vi "Autonomous Independent.vi"   [LabVIEW 2019]
doc: "This VI is called when autonomous begins, and will automatically be terminated when autonomous ends. You can carry out timed or sensor driven robot movement independently without needing to return to the caller."
uses:
  <vilib>/Rock Robotics/WPI/Utilities/WPI_GetSetVariantRefNum.vi
  <vilib>/Rock Robotics/Network Tables/NT Read String.vi
  <vilib>/Rock Robotics/Network Tables/NT Write Numeric Array.vi
  Robot Global Data.vi
panel:
  # "Be sure to right-click and choose Data Operations>>Make Current Value default if you want to save the array values with the VI"
types:
  T1 = typedef "WPI_JoystickDevRef.ctl" = cluster{"Device":T2}
  T2 = typedef "WPI_JoystickDeviceEnum.ctl" = enum16{"USB 0", "USB 1", "USB 2", "USB 3", "USB 4", "USB 5"}
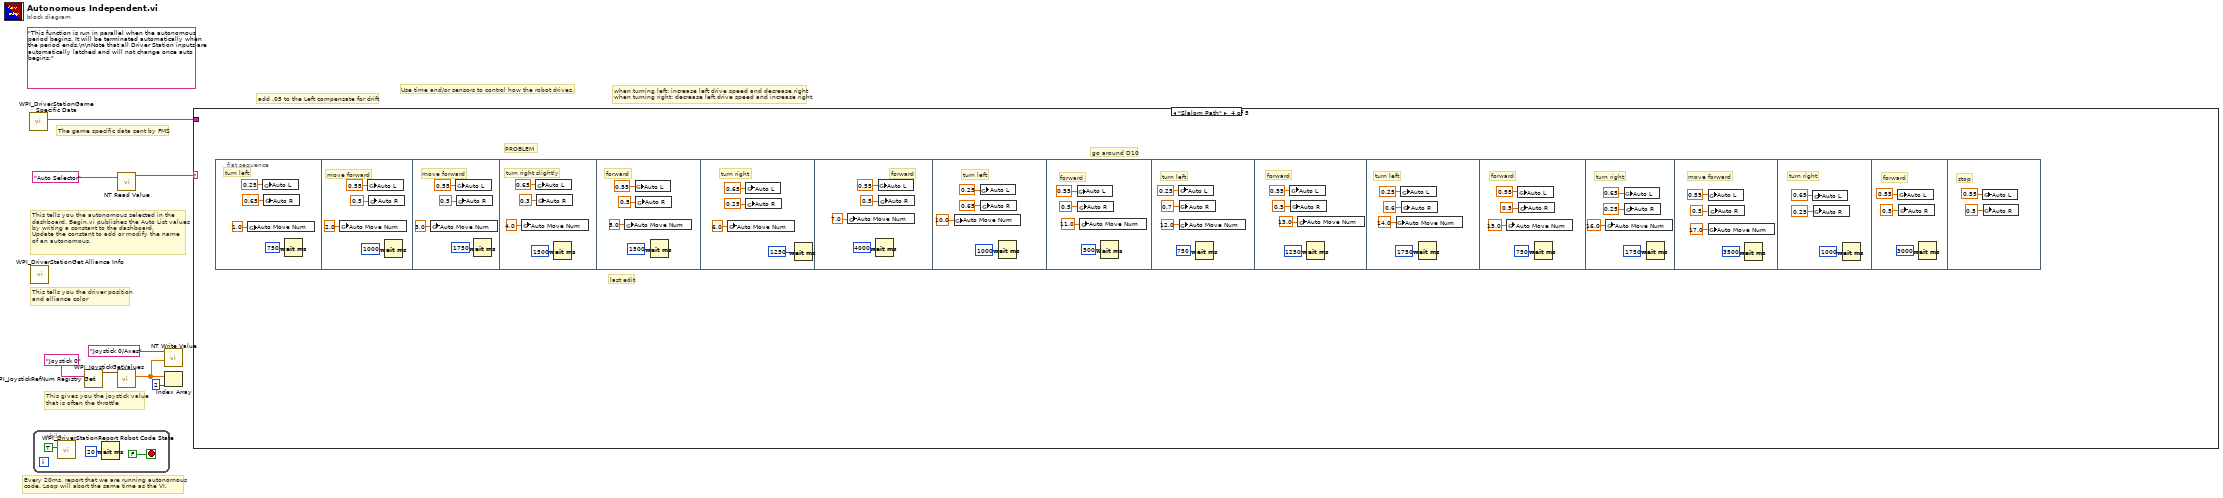
[diagram p0: block diagram]
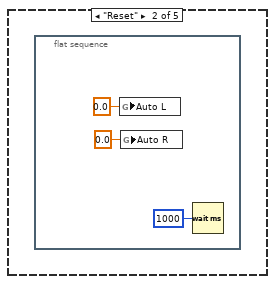
[diagram p3: hidden frame]
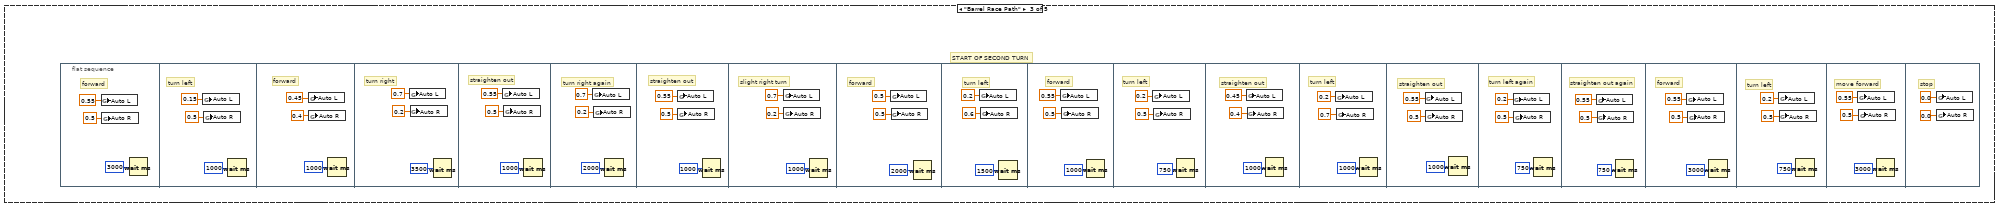
[diagram p4: hidden frame]
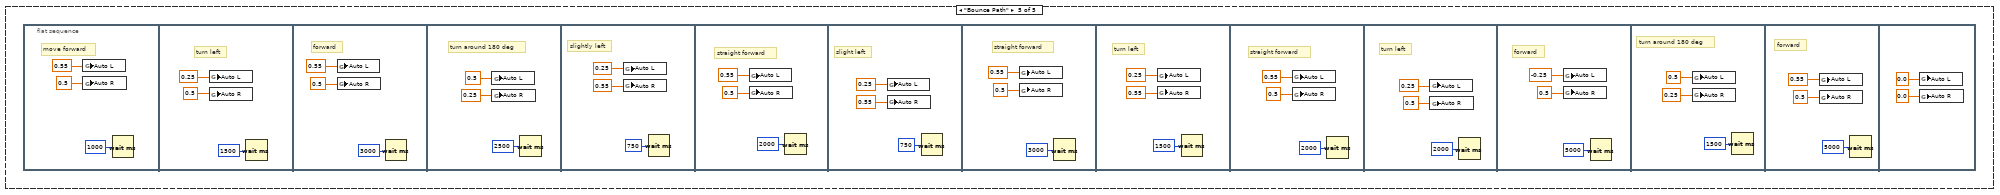
[diagram p5: hidden frame]
diagram:
  (unwired) "This function is run in parallel when the autonomous period begins. It will be terminated automatically when the period ends.\n\nNote that all Driver Station inputs are automatically latched and will not change once auto begins."
  # "add .05 to the Left compensate for drift"
  # "when turning left: increase left drive speed and decrease right\nwhen turning right: decrease left drive speed and increase right"
  # "The game specific data sent by FMS"
  # "This tells you the autonomous selected in the \ndashboard. Begin.vi publishes the Auto List values\nby writing a constant to the dashboard.\nUpdate the constant to add or modify the name\nof an autonomous."
  # "Every 20ms, report that we are running autonomous\ncode. Loop will abort the same time as the VI."
  # "This gives you the joystick value\nthat is often the throttle"
  # "Use time and/or sensors to control how the robot drives."
  # "This tells you the driver position\nand alliance color"
  n1 = call <vilib>:"WPI_DriverStationGame Specific Data.vi"() -> ("Game Specific Data"=w1:string)  [unwired: 11 in]
  n2 = call <vilib>:"WPI_DriverStationGet Alliance Info.vi"() -> ()  [unwired: 12 out]
  n3 = while {
    stop <- FALSE stop-if-true
    n4 = call <vilib>:"WPI_DriverStationReport Robot Code State.vi"("Autonomous"=TRUE) -> ()  [unwired: 10 in, 1 out]
    n5 = Wait (ms)(milliseconds to wait=u32 20) -> ()  [unwired: 1 out]
  }
  n6 = call <vilib>:"WPI_JoystickRefNum Registry Get.vi"("refnum name"="Joystick 0") -> ("JoystickDevRef"=w7:T1)  [unwired: 1 in, 9 out]
  n7 = call <vilib>:"WPI_JoystickGetValues.vi"("JoystickDevRef"=w7) -> ("Axes"=w3:dbl[])  [unwired: 6 in, 4 out]
  n8 = call-poly <vilib>:"NT Read Value.vi"("Name"="Auto Selector") -> ("String"=w4:string)  [unwired: 9 in, 1 out]
  n9 = call-poly <vilib>:"NT Write Value.vi"("Numeric Array"=w3, "Name"="Joystick 0/Axes") -> ()  [unwired: 9 in, 1 out]
  n10 = Index Array(array=w3, index=2) -> ()  [unwired: 1 out]
  n11 = case shown="\"Slalom Path\"" w4 {
    tunnel: w1 -> [_ _ _ _ _]
    frame Default {
      # "You can put your main auto here, or you can right-click on the case and make any\nother frame be the default case."
      # "This is the frame that will execute if no selection is made, or if it is not recognized"
    }
    frame "Reset" {
      n12 = flat-sequence {
        frame #0 {
          n13 = global write "Robot Global Data.vi" "Auto L"(0.0 ("Auto L")) -> ()
          n14 = global write "Robot Global Data.vi" "Auto R"(0.0 ("Auto R")) -> ()
          n15 = Wait (ms)(milliseconds to wait=u32 1000) -> ()  [unwired: 1 out]
        }
      }
    }
    frame "Barrel Race Path" {
      # "START OF SECOND TURN"
      n16 = flat-sequence {
        frame #0 {
          # "forward"
          n17 = global write "Robot Global Data.vi" "Auto L"(0.55 ("Auto X")) -> ()
          n18 = global write "Robot Global Data.vi" "Auto R"(0.5 ("Auto Y")) -> ()
          n19 = Wait (ms)(milliseconds to wait=u32 3000) -> ()  [unwired: 1 out]
        }
        frame #1 {
          # "turn left"
          n20 = global write "Robot Global Data.vi" "Auto L"(0.15 ("Auto X")) -> ()
          n21 = global write "Robot Global Data.vi" "Auto R"(0.5 ("Auto Y")) -> ()
          n22 = Wait (ms)(milliseconds to wait=u32 1000) -> ()  [unwired: 1 out]
        }
        frame #2 {
          # "forward"
          n23 = global write "Robot Global Data.vi" "Auto L"(0.45 ("Auto X")) -> ()
          n24 = global write "Robot Global Data.vi" "Auto R"(0.4 ("Auto Y")) -> ()
          n25 = Wait (ms)(milliseconds to wait=u32 1000) -> ()  [unwired: 1 out]
        }
        frame #3 {
          # "turn right"
          n26 = global write "Robot Global Data.vi" "Auto L"(0.7 ("Auto X")) -> ()
          n27 = global write "Robot Global Data.vi" "Auto R"(0.2 ("Auto Y")) -> ()
          n28 = Wait (ms)(milliseconds to wait=u32 3500) -> ()  [unwired: 1 out]
        }
        frame #4 {
          # "straighten out"
          n29 = global write "Robot Global Data.vi" "Auto L"(0.55 ("Auto X")) -> ()
          n30 = global write "Robot Global Data.vi" "Auto R"(0.5 ("Auto Y")) -> ()
          n31 = Wait (ms)(milliseconds to wait=u32 1000) -> ()  [unwired: 1 out]
        }
        frame #5 {
          # "turn right again"
          n32 = global write "Robot Global Data.vi" "Auto L"(0.7 ("Auto X")) -> ()
          n33 = global write "Robot Global Data.vi" "Auto R"(0.2 ("Auto Y")) -> ()
          n34 = Wait (ms)(milliseconds to wait=u32 2000) -> ()  [unwired: 1 out]
        }
        frame #6 {
          # "straighten out"
          n35 = global write "Robot Global Data.vi" "Auto L"(0.55 ("Auto X")) -> ()
          n36 = global write "Robot Global Data.vi" "Auto R"(0.5 ("Auto Y")) -> ()
          n37 = Wait (ms)(milliseconds to wait=u32 1000) -> ()  [unwired: 1 out]
        }
        frame #7 {
          # "slight right turn"
          n38 = global write "Robot Global Data.vi" "Auto L"(0.7 ("Auto X")) -> ()
          n39 = global write "Robot Global Data.vi" "Auto R"(0.2 ("Auto Y")) -> ()
          n40 = Wait (ms)(milliseconds to wait=u32 1000) -> ()  [unwired: 1 out]
        }
        frame #8 {
          # "forward"
          n41 = global write "Robot Global Data.vi" "Auto L"(0.5 ("Auto X")) -> ()
          n42 = global write "Robot Global Data.vi" "Auto R"(0.5 ("Auto Y")) -> ()
          n43 = Wait (ms)(milliseconds to wait=u32 2000) -> ()  [unwired: 1 out]
        }
        frame #9 {
          # "turn left"
          n44 = global write "Robot Global Data.vi" "Auto L"(0.2 ("Auto X")) -> ()
          n45 = global write "Robot Global Data.vi" "Auto R"(0.6 ("Auto Y")) -> ()
          n46 = Wait (ms)(milliseconds to wait=u32 1500) -> ()  [unwired: 1 out]
        }
        frame #10 {
          # "forward"
          n47 = global write "Robot Global Data.vi" "Auto L"(0.55 ("Auto X")) -> ()
          n48 = global write "Robot Global Data.vi" "Auto R"(0.5 ("Auto Y")) -> ()
          n49 = Wait (ms)(milliseconds to wait=u32 1000) -> ()  [unwired: 1 out]
        }
        frame #11 {
          # "turn left"
          n50 = global write "Robot Global Data.vi" "Auto L"(0.2 ("Auto X")) -> ()
          n51 = global write "Robot Global Data.vi" "Auto R"(0.5 ("Auto Y")) -> ()
          n52 = Wait (ms)(milliseconds to wait=u32 750) -> ()  [unwired: 1 out]
        }
        frame #12 {
          # "straighten out"
          n53 = global write "Robot Global Data.vi" "Auto L"(0.45 ("Auto X")) -> ()
          n54 = global write "Robot Global Data.vi" "Auto R"(0.4 ("Auto Y")) -> ()
          n55 = Wait (ms)(milliseconds to wait=u32 1000) -> ()  [unwired: 1 out]
        }
        frame #13 {
          # "turn left"
          n56 = global write "Robot Global Data.vi" "Auto L"(0.2 ("Auto X")) -> ()
          n57 = global write "Robot Global Data.vi" "Auto R"(0.7 ("Auto Y")) -> ()
          n58 = Wait (ms)(milliseconds to wait=u32 1000) -> ()  [unwired: 1 out]
        }
        frame #14 {
          # "straighten out"
          n59 = global write "Robot Global Data.vi" "Auto L"(0.55 ("Auto X")) -> ()
          n60 = global write "Robot Global Data.vi" "Auto R"(0.5 ("Auto Y")) -> ()
          n61 = Wait (ms)(milliseconds to wait=u32 1000) -> ()  [unwired: 1 out]
        }
        frame #15 {
          # "turn left again"
          n62 = global write "Robot Global Data.vi" "Auto L"(0.2 ("Auto X")) -> ()
          n63 = global write "Robot Global Data.vi" "Auto R"(0.5 ("Auto Y")) -> ()
          n64 = Wait (ms)(milliseconds to wait=u32 750) -> ()  [unwired: 1 out]
        }
        frame #16 {
          # "straighten out again"
          n65 = global write "Robot Global Data.vi" "Auto L"(0.55 ("Auto X")) -> ()
          n66 = global write "Robot Global Data.vi" "Auto R"(0.5 ("Auto Y")) -> ()
          n67 = Wait (ms)(milliseconds to wait=u32 750) -> ()  [unwired: 1 out]
        }
        frame #17 {
          # "forward"
          n68 = global write "Robot Global Data.vi" "Auto L"(0.55 ("Auto X")) -> ()
          n69 = global write "Robot Global Data.vi" "Auto R"(0.5 ("Auto Y")) -> ()
          n70 = Wait (ms)(milliseconds to wait=u32 3000) -> ()  [unwired: 1 out]
        }
        frame #18 {
          # "turn left"
          n71 = global write "Robot Global Data.vi" "Auto L"(0.2 ("Auto X")) -> ()
          n72 = global write "Robot Global Data.vi" "Auto R"(0.5 ("Auto Y")) -> ()
          n73 = Wait (ms)(milliseconds to wait=u32 750) -> ()  [unwired: 1 out]
        }
        frame #19 {
          # "move forward"
          n74 = global write "Robot Global Data.vi" "Auto L"(0.55 ("Auto X")) -> ()
          n75 = global write "Robot Global Data.vi" "Auto R"(0.5 ("Auto Y")) -> ()
          n76 = Wait (ms)(milliseconds to wait=u32 3000) -> ()  [unwired: 1 out]
        }
        frame #20 {
          # "stop"
          n77 = global write "Robot Global Data.vi" "Auto L"(0.0 ("Auto X")) -> ()
          n78 = global write "Robot Global Data.vi" "Auto R"(0.0 ("Auto Y")) -> ()
        }
      }
    }
    frame "Slalom Path" {
      # "last edit"
      # "PROBLEM"
      # "go around D10"
      n79 = flat-sequence {
        frame #0 {
          # "turn left"
          n80 = global write "Robot Global Data.vi" "Auto Move Num"(1.0 ("Auto Move Num")) -> ()
          n81 = global write "Robot Global Data.vi" "Auto L"(0.25 ("Auto L")) -> ()
          n82 = global write "Robot Global Data.vi" "Auto R"(0.65 ("Auto R")) -> ()
          n83 = Wait (ms)(milliseconds to wait=u32 750) -> ()  [unwired: 1 out]
        }
        frame #1 {
          # "move forward"
          n84 = global write "Robot Global Data.vi" "Auto Move Num"(2.0 ("Auto Move Num")) -> ()
          n85 = global write "Robot Global Data.vi" "Auto L"(0.55 ("Auto L")) -> ()
          n86 = global write "Robot Global Data.vi" "Auto R"(0.5 ("Auto R")) -> ()
          n87 = Wait (ms)(milliseconds to wait=u32 1000) -> ()  [unwired: 1 out]
        }
        frame #2 {
          # "move forward"
          n88 = global write "Robot Global Data.vi" "Auto Move Num"(3.0 ("Auto Move Num")) -> ()
          n89 = global write "Robot Global Data.vi" "Auto L"(0.55 ("Auto L")) -> ()
          n90 = global write "Robot Global Data.vi" "Auto R"(0.5 ("Auto R")) -> ()
          n91 = Wait (ms)(milliseconds to wait=u32 1750) -> ()  [unwired: 1 out]
        }
        frame #3 {
          # "turn right slightly"
          n92 = global write "Robot Global Data.vi" "Auto Move Num"(4.0 ("Auto Move Num")) -> ()
          n93 = global write "Robot Global Data.vi" "Auto L"(0.65 ("Auto L")) -> ()
          n94 = global write "Robot Global Data.vi" "Auto R"(0.3 ("Auto R")) -> ()
          n95 = Wait (ms)(milliseconds to wait=u32 1500) -> ()  [unwired: 1 out]
        }
        frame #4 {
          # "forward"
          n96 = global write "Robot Global Data.vi" "Auto Move Num"(5.0 ("Auto Move Num")) -> ()
          n97 = global write "Robot Global Data.vi" "Auto L"(0.55 ("Auto L")) -> ()
          n98 = global write "Robot Global Data.vi" "Auto R"(0.5 ("Auto R")) -> ()
          n99 = Wait (ms)(milliseconds to wait=u32 1500) -> ()  [unwired: 1 out]
        }
        frame #5 {
          # "turn right"
          n100 = global write "Robot Global Data.vi" "Auto Move Num"(6.0 ("Auto Move Num")) -> ()
          n101 = global write "Robot Global Data.vi" "Auto L"(0.65 ("Auto L")) -> ()
          n102 = global write "Robot Global Data.vi" "Auto R"(0.25 ("Auto R")) -> ()
          n103 = Wait (ms)(milliseconds to wait=u32 1250) -> ()  [unwired: 1 out]
        }
        frame #6 {
          # "forward"
          n104 = global write "Robot Global Data.vi" "Auto Move Num"(7.0 ("Auto Move Num")) -> ()
          n105 = Wait (ms)(milliseconds to wait=u32 4000) -> ()  [unwired: 1 out]
          n106 = global write "Robot Global Data.vi" "Auto L"(0.55 ("Auto L")) -> ()
          n107 = global write "Robot Global Data.vi" "Auto R"(0.5 ("Auto R")) -> ()
        }
        frame #7 {
          # "turn left"
          n108 = global write "Robot Global Data.vi" "Auto Move Num"(10.0 ("Auto Move Num")) -> ()
          n109 = global write "Robot Global Data.vi" "Auto L"(0.25 ("Auto L")) -> ()
          n110 = global write "Robot Global Data.vi" "Auto R"(0.65 ("Auto R")) -> ()
          n111 = Wait (ms)(milliseconds to wait=u32 1000) -> ()  [unwired: 1 out]
        }
        frame #8 {
          # "forward"
          n112 = global write "Robot Global Data.vi" "Auto L"(0.55 ("Auto L")) -> ()
          n113 = global write "Robot Global Data.vi" "Auto R"(0.5 ("Auto R")) -> ()
          n114 = global write "Robot Global Data.vi" "Auto Move Num"(11.0 ("Auto Move Num")) -> ()
          n115 = Wait (ms)(milliseconds to wait=u32 500) -> ()  [unwired: 1 out]
        }
        frame #9 {
          # "turn left"
          n116 = global write "Robot Global Data.vi" "Auto L"(0.25 ("Auto L")) -> ()
          n117 = global write "Robot Global Data.vi" "Auto R"(0.7 ("Auto R")) -> ()
          n118 = global write "Robot Global Data.vi" "Auto Move Num"(12.0 ("Auto Move Num")) -> ()
          n119 = Wait (ms)(milliseconds to wait=u32 750) -> ()  [unwired: 1 out]
        }
        frame #10 {
          # "forward"
          n120 = global write "Robot Global Data.vi" "Auto L"(0.55 ("Auto L")) -> ()
          n121 = global write "Robot Global Data.vi" "Auto R"(0.5 ("Auto R")) -> ()
          n122 = global write "Robot Global Data.vi" "Auto Move Num"(13.0 ("Auto Move Num")) -> ()
          n123 = Wait (ms)(milliseconds to wait=u32 1250) -> ()  [unwired: 1 out]
        }
        frame #11 {
          # "turn left"
          n124 = global write "Robot Global Data.vi" "Auto Move Num"(14.0 ("Auto Move Num")) -> ()
          n125 = global write "Robot Global Data.vi" "Auto L"(0.25 ("Auto L")) -> ()
          n126 = global write "Robot Global Data.vi" "Auto R"(0.6 ("Auto R")) -> ()
          n127 = Wait (ms)(milliseconds to wait=u32 1750) -> ()  [unwired: 1 out]
        }
        frame #12 {
          # "forward"
          n128 = global write "Robot Global Data.vi" "Auto Move Num"(15.0 ("Auto Move Num")) -> ()
          n129 = global write "Robot Global Data.vi" "Auto L"(0.55 ("Auto L")) -> ()
          n130 = global write "Robot Global Data.vi" "Auto R"(0.5 ("Auto R")) -> ()
          n131 = Wait (ms)(milliseconds to wait=u32 750) -> ()  [unwired: 1 out]
        }
        frame #13 {
          # "turn right"
          n132 = global write "Robot Global Data.vi" "Auto Move Num"(16.0 ("Auto Move Num")) -> ()
          n133 = global write "Robot Global Data.vi" "Auto L"(0.65 ("Auto L")) -> ()
          n134 = global write "Robot Global Data.vi" "Auto R"(0.25 ("Auto R")) -> ()
          n135 = Wait (ms)(milliseconds to wait=u32 1750) -> ()  [unwired: 1 out]
        }
        frame #14 {
          # "move forward"
          n136 = global write "Robot Global Data.vi" "Auto L"(0.55 ("Auto L")) -> ()
          n137 = global write "Robot Global Data.vi" "Auto Move Num"(17.0 ("Auto Move Num")) -> ()
          n138 = global write "Robot Global Data.vi" "Auto R"(0.5 ("Auto R")) -> ()
          n139 = Wait (ms)(milliseconds to wait=u32 3500) -> ()  [unwired: 1 out]
        }
        frame #15 {
          # "turn right"
          n140 = global write "Robot Global Data.vi" "Auto L"(0.65 ("Auto L")) -> ()
          n141 = global write "Robot Global Data.vi" "Auto R"(0.25 ("Auto R")) -> ()
          n142 = Wait (ms)(milliseconds to wait=u32 1000) -> ()  [unwired: 1 out]
        }
        frame #16 {
          # "forward"
          n143 = global write "Robot Global Data.vi" "Auto L"(0.55 ("Auto L")) -> ()
          n144 = global write "Robot Global Data.vi" "Auto R"(0.5 ("Auto R")) -> ()
          n145 = Wait (ms)(milliseconds to wait=u32 3000) -> ()  [unwired: 1 out]
        }
        frame #17 {
          # "stop"
          n146 = global write "Robot Global Data.vi" "Auto L"(0.55 ("Auto L")) -> ()
          n147 = global write "Robot Global Data.vi" "Auto R"(0.5 ("Auto R")) -> ()
        }
      }
    }
    frame "Bounce Path" {
      n148 = flat-sequence {
        frame #0 {
          # "move forward"
          n149 = global write "Robot Global Data.vi" "Auto L"(0.55 ("Joystick X")) -> ()
          n150 = global write "Robot Global Data.vi" "Auto R"(0.5 ("Joystick Y")) -> ()
          n151 = Wait (ms)(milliseconds to wait=u32 1000) -> ()  [unwired: 1 out]
        }
        frame #1 {
          # "turn left"
          n152 = global write "Robot Global Data.vi" "Auto L"(0.25 ("Joystick X")) -> ()
          n153 = global write "Robot Global Data.vi" "Auto R"(0.5 ("Joystick Y")) -> ()
          n154 = Wait (ms)(milliseconds to wait=u32 1500) -> ()  [unwired: 1 out]
        }
        frame #2 {
          # "forward"
          n155 = global write "Robot Global Data.vi" "Auto L"(0.55 ("Joystick X")) -> ()
          n156 = global write "Robot Global Data.vi" "Auto R"(0.5 ("Joystick Y")) -> ()
          n157 = Wait (ms)(milliseconds to wait=u32 3000) -> ()  [unwired: 1 out]
        }
        frame #3 {
          # "turn around 180 deg"
          n158 = global write "Robot Global Data.vi" "Auto L"(0.5 ("Joystick X")) -> ()
          n159 = global write "Robot Global Data.vi" "Auto R"(0.25 ("Joystick Y")) -> ()
          n160 = Wait (ms)(milliseconds to wait=u32 2500) -> ()  [unwired: 1 out]
        }
        frame #4 {
          # "slightly left"
          n161 = global write "Robot Global Data.vi" "Auto L"(0.25 ("Joystick X")) -> ()
          n162 = global write "Robot Global Data.vi" "Auto R"(0.55 ("Joystick Y")) -> ()
          n163 = Wait (ms)(milliseconds to wait=u32 750) -> ()  [unwired: 1 out]
        }
        frame #5 {
          # "straight forward"
          n164 = global write "Robot Global Data.vi" "Auto L"(0.55 ("Joystick X")) -> ()
          n165 = global write "Robot Global Data.vi" "Auto R"(0.5 ("Joystick Y")) -> ()
          n166 = Wait (ms)(milliseconds to wait=u32 2000) -> ()  [unwired: 1 out]
        }
        frame #6 {
          # "slight left"
          n167 = global write "Robot Global Data.vi" "Auto L"(0.25 ("Joystick X")) -> ()
          n168 = global write "Robot Global Data.vi" "Auto R"(0.55 ("Joystick Y")) -> ()
          n169 = Wait (ms)(milliseconds to wait=u32 750) -> ()  [unwired: 1 out]
        }
        frame #7 {
          # "straight forward"
          n170 = global write "Robot Global Data.vi" "Auto L"(0.55 ("Joystick X")) -> ()
          n171 = global write "Robot Global Data.vi" "Auto R"(0.5 ("Joystick Y")) -> ()
          n172 = Wait (ms)(milliseconds to wait=u32 3000) -> ()  [unwired: 1 out]
        }
        frame #8 {
          # "turn left"
          n173 = global write "Robot Global Data.vi" "Auto L"(0.25 ("Joystick X")) -> ()
          n174 = global write "Robot Global Data.vi" "Auto R"(0.55 ("Joystick Y")) -> ()
          n175 = Wait (ms)(milliseconds to wait=u32 1500) -> ()  [unwired: 1 out]
        }
        frame #9 {
          # "straight forward"
          n176 = global write "Robot Global Data.vi" "Auto L"(0.55 ("Joystick X")) -> ()
          n177 = global write "Robot Global Data.vi" "Auto R"(0.5 ("Joystick Y")) -> ()
          n178 = Wait (ms)(milliseconds to wait=u32 2000) -> ()  [unwired: 1 out]
        }
        frame #10 {
          # "turn left"
          n179 = global write "Robot Global Data.vi" "Auto L"(0.25 ("Joystick X")) -> ()
          n180 = global write "Robot Global Data.vi" "Auto R"(0.5 ("Joystick Y")) -> ()
          n181 = Wait (ms)(milliseconds to wait=u32 2000) -> ()  [unwired: 1 out]
        }
        frame #11 {
          # "forward"
          n182 = global write "Robot Global Data.vi" "Auto L"(-0.25 ("Joystick X")) -> ()
          n183 = global write "Robot Global Data.vi" "Auto R"(0.5 ("Joystick Y")) -> ()
          n184 = Wait (ms)(milliseconds to wait=u32 5000) -> ()  [unwired: 1 out]
        }
        frame #12 {
          # "turn around 180 deg"
          n185 = global write "Robot Global Data.vi" "Auto L"(0.5 ("Joystick X")) -> ()
          n186 = global write "Robot Global Data.vi" "Auto R"(0.25 ("Joystick Y")) -> ()
          n187 = Wait (ms)(milliseconds to wait=u32 1500) -> ()  [unwired: 1 out]
        }
        frame #13 {
          # "forward"
          n188 = global write "Robot Global Data.vi" "Auto L"(0.55 ("Joystick X")) -> ()
          n189 = global write "Robot Global Data.vi" "Auto R"(0.5 ("Joystick Y")) -> ()
          n190 = Wait (ms)(milliseconds to wait=u32 5000) -> ()  [unwired: 1 out]
        }
        frame #14 {
          n191 = global write "Robot Global Data.vi" "Auto L"(0.0 ("Joystick X")) -> ()
          n192 = global write "Robot Global Data.vi" "Auto R"(0.0 ("Joystick Y")) -> ()
        }
      }
    }
  }
